vi "DriveStateController.vi"(1 "Selected State (In)":string) -> (0 "Selected State (Out)":string)   [LabVIEW 2019]
uses:
  <vilib>/Rock Robotics/WPI/DriverStation/WPI_DriverStationRobotMode2.ctl
  sensors.vi
  dsinstructions.vi
  dsdata.vi
  outputs.vi
  constants.vi
panel:
  in  "Rotation Scaling":dbl[](array[slide])=[3.0, 2.0, 4.0, 1.0] min=1.0 max=4.0 scale=1.0..4.0
  in  "Strafe Scaling":dbl[](array[slide])=[3.0, 2.0, 4.0, 1.0] min=1.0 max=4.0 scale=1.0..4.0
  in  "Rotation Deadband":dbl[](array[slide])=[0.05, 0.2, 0.2, 0.0] min=0.0 max=1.0 scale=0.0..1.0
  in  "Strafe Deadband":dbl[](array[slide])=[0.05, 0.2, 0.2, 0.0] min=0.0 max=1.0 scale=0.0..1.0
  in  "Sync Driver Profile":bool
  out "Current_Driver":string
  in  "Zero Wheels":bool
  in  "Hysteresis (deg)":dbl=20.0 format="%#_13g"
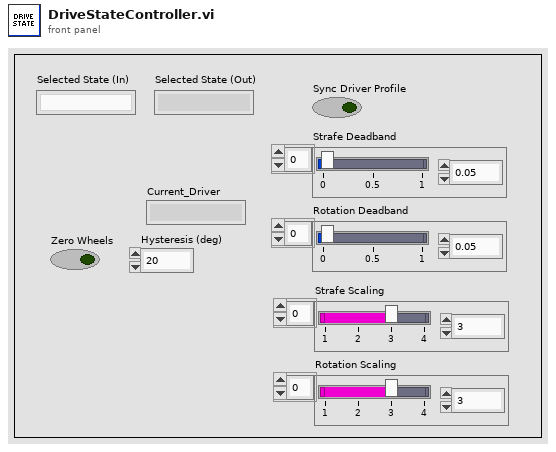
[diagram p1: front panel]
types:
  T1 = typedef "WPI_DriverStationRobotMode2.ctl" = enum16{"Autonomous Disabled", "Autonomous Enabled", "Teleop Disabled", "Teleop Enabled", "Disconnected", "Finish", "Test Disabled", "Test Enabled", "Emergency Stopped"}
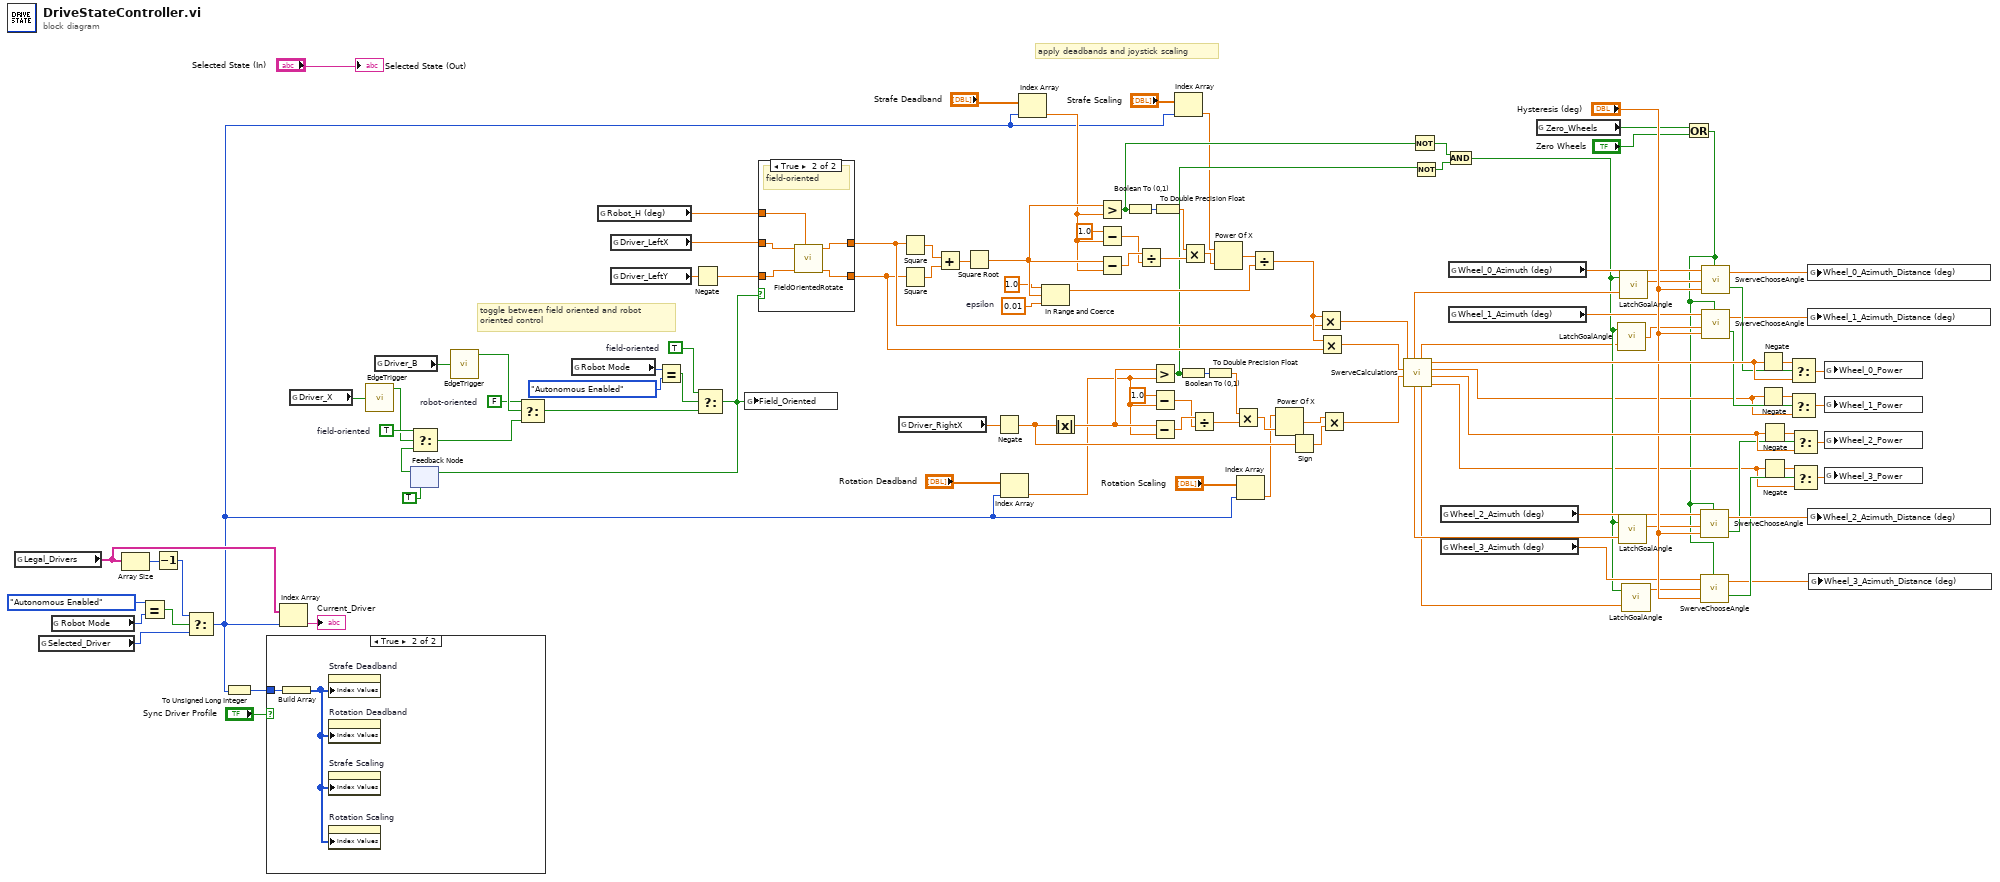
[diagram p0: block diagram]
diagram:
  w13 = TRUE  # field-oriented
  w59 = TRUE  # field-oriented
  w60 = FALSE  # robot-oriented
  w79 = 0.01  # epsilon
  # "apply deadbands and joystick scaling"
  # "toggle between field oriented and robot \noriented control"
  n1 = global read "constants.vi" "Legal_Drivers"() -> (w2:string[])
  n2 = global read "dsdata.vi" "Selected_Driver"() -> (w5:i32)
  n3 = global read "dsdata.vi" "Robot Mode"() -> (w8:T1)
  n4 = Array Size(array=w2) -> (size(s)=w4:i32)
  n5 = Equal?(x=WPI_DriverStationRobotMode2."Autonomous Enabled", y=w8) -> (x = y?=w6:bool)
  n6 = Decrement(x=w4) -> (x-1=w3:i32)
  n7 = Select(t=w3, s=w6, f=w5) -> (s? t:f=w1:i32)
  n8 = To Unsigned Long Integer(number=w1) -> (unsigned 32bit integer=w29:u32)
  n9 = case shown="True" "Sync Driver Profile" {
    tunnel: w29 -> [_ w115]
    frame False {
    }
    frame True {
      n10 = Build Array(w115) -> (w114:u32[])
      n11 = property on="Strafe Deadband" class="Arr (strict)"("Index Values"=w114) -> ()  [unwired: 2 in, 2 out]
      n12 = property on="Rotation Deadband" class="Arr (strict)"("Index Values"=w114) -> ()  [unwired: 2 in, 2 out]
      n13 = property on="Strafe Scaling" class="Arr (strict)"("Index Values"=w114) -> ()  [unwired: 2 in, 2 out]
      n14 = property on="Rotation Scaling" class="Arr (strict)"("Index Values"=w114) -> ()  [unwired: 2 in, 2 out]
    }
  }
  n15 = Index Array(array=w2, index=w1) -> (element=→"Current_Driver":string)
  n16 = global read "dsinstructions.vi" "Driver_X"() -> (w63:bool)
  n17 = call "EdgeTrigger.vi"("Input Signal"=w63) -> ("Rising Edge Trigger"=w39:bool)  [unwired: 2 out]
  n18 = global read "dsinstructions.vi" "Driver_B"() -> (w64:bool)
  n19 = feedback #1(TRUE) -> (w57:bool)
  n20 = Select(t=w59, s=w39, f=w57) -> (s? t:f=w58:bool)
  n21 = call "EdgeTrigger.vi"("Input Signal"=w64) -> ("Rising Edge Trigger"=w61:bool)  [unwired: 2 out]
  n22 = Select(t=w60, s=w61, f=w58) -> (s? t:f=w15:bool)
  n23 = global read "dsdata.vi" "Robot Mode"() -> (w12:T1)
  n24 = global read "sensors.vi" "Robot_H (deg)"() -> (w56:dbl)
  n25 = global read "dsinstructions.vi" "Driver_LeftX"() -> (w52:dbl)
  n26 = global read "dsinstructions.vi" "Driver_LeftY"() -> (w82:dbl)
  n27 = Equal?(x=w12, y=WPI_DriverStationRobotMode2."Autonomous Enabled") -> (x = y?=w10:bool)
  n28 = Negate(x=w82) -> (-x=w66:dbl)
  n29 = Select(t=w13, s=w10, f=w15) -> (s? t:f=w14:bool)
  n30 = feedback-in #1(w14) -> ()
  n31 = global write "outputs.vi" "Field_Oriented"(w14) -> ()
  n32 = case shown="True" w14 {
    tunnel: [w117 w122] -> w67
    tunnel: w52 -> [w117 w120]
    tunnel: [w116 w121] -> w65
    tunnel: w66 -> [w116 w119]
    tunnel: w56 -> [_ w118]
    frame False {
      # "robot-oriented"
    }
    frame True {
      # "field-oriented"
      n33 = call "FieldOrientedRotate.vi"("Angle (deg)"=w118, "Y"=w119, "X"=w120) -> ("Y'"=w121:dbl, "X'"=w122:dbl)  [unwired: 7 in]
    }
  }
  n34 = global read "dsinstructions.vi" "Driver_RightX"() -> (w40:dbl)
  n35 = Square(x=w67) -> (x^2=w83:dbl)
  n36 = Square(x=w65) -> (x^2=w84:dbl)
  n37 = Add(x=w83, y=w84) -> (x+y=w81:dbl)
  n38 = Square Root(x=w81) -> (sqrt(x)=w78:dbl)
  n39 = Negate(x=w40) -> (-x=w31:dbl)
  n40 = Index Array(array="Rotation Deadband", index=w1) -> (element=w24:dbl)
  n41 = Index Array(array="Strafe Deadband", index=w1) -> (element=w27:dbl)
  n42 = In Range and Coerce(upper limit=1.0, x=w78, lower limit=w79) -> (coerced(x)=w80:dbl)  [unwired: 1 out]
  n43 = Absolute Value(x=w31) -> (abs(x)=w53:dbl)
  n44 = Greater?(x=w78, y=w27) -> (0:w49:bool)
  n45 = Subtract(x=1.0, y=w27) -> (x-y=w86:dbl)
  n46 = Subtract(x=w78, y=w27) -> (x-y=w88:dbl)
  n47 = Boolean To (0,1)(Boolean=w49) -> (0, 1=w90:i16)
  n48 = Divide(x=w88, y=w86) -> (x/y=w85:dbl)
  n49 = Greater?(x=w53, y=w24) -> (0:w48:bool)
  n50 = Subtract(x=1.0, y=w24) -> (x-y=w69:dbl)
  n51 = Subtract(x=w53, y=w24) -> (x-y=w71:dbl)
  n52 = To Double Precision Float(number=w90) -> (double precision float=w89:dbl)
  n53 = Index Array(array="Strafe Scaling", index=w1) -> (element=w16:dbl)
  n54 = Boolean To (0,1)(Boolean=w48) -> (0, 1=w73:i16)
  n55 = Multiply(x=w89, y=w85) -> (x*y=w18:dbl)
  n56 = Divide(x=w71, y=w69) -> (x/y=w68:dbl)
  n57 = To Double Precision Float(number=w73) -> (double precision float=w72:dbl)
  n58 = Power Of X(1:w18, 2:w16) -> (0:w17:dbl)
  n59 = Multiply(x=w72, y=w68) -> (x*y=w22:dbl)
  n60 = Index Array(array="Rotation Scaling", index=w1) -> (element=w20:dbl)
  n61 = Divide(x=w17, y=w80) -> (x/y=w76:dbl)
  n62 = Power Of X(1:w22, 2:w20) -> (0:w21:dbl)
  n63 = Sign(1:w31) -> (0:w54:dbl)
  n64 = Multiply(x=w76, y=w67) -> (x*y=w75:dbl)
  n65 = Multiply(x=w76, y=w65) -> (x*y=w74:dbl)
  n66 = Multiply(x=w21, y=w54) -> (x*y=w55:dbl)
  n67 = call "SwerveCalculations.vi"("J2X"=w55, "J1Y"=w74, "J1X"=w75) -> ("Magnitude 3"=w35:dbl, "Magnitude 2"=w111:dbl, "Magnitude 1"=w37:dbl, "Magnitude 0"=w110:dbl, "Wheel Angle 3"=w36:dbl, "Wheel Angle 1"=w38:dbl, "Wheel Angle 2"=w44:dbl, "Wheel Angle 0"=w51:dbl)  [unwired: 1 in]
  n68 = Not(x=w49) -> (.not. x?=w46:bool)
  n69 = Not(x=w48) -> (.not. x?=w47:bool)
  n70 = global read "sensors.vi" "Wheel_2_Azimuth (deg)"() -> (w105:dbl)
  n71 = global read "sensors.vi" "Wheel_3_Azimuth (deg)"() -> (w91:dbl)
  n72 = And(x=w46, y=w47) -> (x .and. y?=w41:bool)
  n73 = global read "sensors.vi" "Wheel_0_Azimuth (deg)"() -> (w93:dbl)
  n74 = global read "sensors.vi" "Wheel_1_Azimuth (deg)"() -> (w92:dbl)
  n75 = global read "dsdata.vi" "Zero_Wheels"() -> (w34:bool)
  n76 = call "LatchGoalAngle.vi"("Raw Goal Angle"=w38, "In Deadband"=w41) -> ("Latched Goal Angle"=w45:dbl)
  n77 = call "LatchGoalAngle.vi"("Raw Goal Angle"=w44, "In Deadband"=w41) -> ("Latched Goal Angle"=w43:dbl)
  n78 = call "LatchGoalAngle.vi"("Raw Goal Angle"=w51, "In Deadband"=w41) -> ("Latched Goal Angle"=w50:dbl)
  n79 = call "LatchGoalAngle.vi"("Raw Goal Angle"=w36, "In Deadband"=w41) -> ("Latched Goal Angle"=w42:dbl)
  n80 = Or(x=w34, y="Zero Wheels") -> (x .or. y?=w33:bool)
  n81 = call "SwerveChooseAngle.vi"("Zero Wheels"=w33, "Hysteresis (deg)"="Hysteresis (deg)", "Goal Angle (deg)"=w43, "Current Angle (deg)"=w105) -> ("Invert Speed  Motor (?)"=w107:bool, "Angular Distance (deg)"=w108:dbl)
  n82 = call "SwerveChooseAngle.vi"("Zero Wheels"=w33, "Hysteresis (deg)"="Hysteresis (deg)", "Goal Angle (deg)"=w42, "Current Angle (deg)"=w91) -> ("Invert Speed  Motor (?)"=w106:bool, "Angular Distance (deg)"=w96:dbl)
  n83 = call "SwerveChooseAngle.vi"("Zero Wheels"=w33, "Hysteresis (deg)"="Hysteresis (deg)", "Goal Angle (deg)"=w50, "Current Angle (deg)"=w93) -> ("Invert Speed  Motor (?)"=w100:bool, "Angular Distance (deg)"=w98:dbl)
  n84 = call "SwerveChooseAngle.vi"("Zero Wheels"=w33, "Hysteresis (deg)"="Hysteresis (deg)", "Goal Angle (deg)"=w45, "Current Angle (deg)"=w92) -> ("Invert Speed  Motor (?)"=w99:bool, "Angular Distance (deg)"=w97:dbl)
  n85 = Negate(x=w110) -> (-x=w104:dbl)
  n86 = Negate(x=w37) -> (-x=w102:dbl)
  n87 = Negate(x=w111) -> (-x=w113:dbl)
  n88 = Negate(x=w35) -> (-x=w95:dbl)
  n89 = Select(t=w104, s=w100, f=w110) -> (s? t:f=w103:dbl)
  n90 = Select(t=w102, s=w99, f=w37) -> (s? t:f=w101:dbl)
  n91 = Select(t=w113, s=w107, f=w111) -> (s? t:f=w112:dbl)
  n92 = Select(t=w95, s=w106, f=w35) -> (s? t:f=w94:dbl)
  n93 = global write "outputs.vi" "Wheel_0_Azimuth_Distance (deg)"(w98) -> ()
  n94 = global write "outputs.vi" "Wheel_1_Azimuth_Distance (deg)"(w97) -> ()
  n95 = global write "outputs.vi" "Wheel_2_Azimuth_Distance (deg)"(w108) -> ()
  n96 = global write "outputs.vi" "Wheel_3_Azimuth_Distance (deg)"(w96) -> ()
  n97 = global write "outputs.vi" "Wheel_0_Power"(w103) -> ()
  n98 = global write "outputs.vi" "Wheel_1_Power"(w101) -> ()
  n99 = global write "outputs.vi" "Wheel_2_Power"(w112) -> ()
  n100 = global write "outputs.vi" "Wheel_3_Power"(w94) -> ()
  "Selected State (Out)" <- "Selected State (In)"
